vi "SolenoidTest.vi"() -> ()   [LabVIEW 2013]
uses:
  <vilib>/Rock Robotics/SystemInterfaces/DIO/FPGA_DIOChannel.ctl
  <vilib>/Rock Robotics/SystemInterfaces/Typedef/FPGA_TypedefDigitalModule.ctl
  <vilib>/Rock Robotics/SystemInterfaces/DIO/FPGA_DIORelayChannel.ctl
  <vilib>/Rock Robotics/WPI/Joystick/WPI_JoystickDeviceEnum.ctl
  <vilib>/Rock Robotics/WPI/Solenoid/WPI_SolenoidChannel.ctl
  Robot_Framework_2014/DoubleSolenoidAction.ctl
  Robot_Framework_2014/SingleSolenoidAction.ctl
  <vilib>/Rock Robotics/WPI/Solenoid/WPI_SolenoidOpenSingle.vi
panel:
  in  "Single?":bool
  # "BUTTON 5\nL1"
  # "BUTTON 6\nR1"
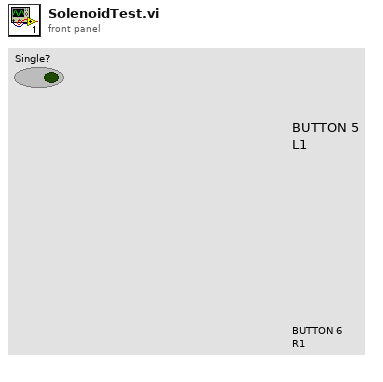
[diagram p1: front panel]
types:
  T1 = typedef "WPI_JoystickDeviceEnum.ctl" = enum16{"USB 1", "USB 2", "USB 3", "USB 4", "Kinect 1", "Kinect 2"}
  T2 = typedef "FPGA_DIORelayChannel.ctl" = enum8{"Relay 1", "Relay 2", "Relay 3", "Relay 4", "Relay 5", "Relay 6", "Relay 7", "Relay 8", "Invalid"}
  T3 = typedef "FPGA_TypedefDigitalModule.ctl" = enum16{"Digital Module 1", "Digital Module 2"}
  T4 = typedef "FPGA_DIOChannel.ctl" = enum8{"DIO 1", "DIO 2", "DIO 3", "DIO 4", "DIO 5", "DIO 6", "DIO 7", "DIO 8", "DIO 9", "DIO 10", "DIO 11", "DIO 12", "DIO 13", "DIO 14", "Invalid"}
  T5 = typedef "WPI_JoystickDevRef.ctl" = cluster{"Device":T1}
  T6 = typedef "DoubleSolenoidAction.ctl" = enum16{"Init", "Middle", "In", "Out"}
  T7 = typedef "WPI_SolenoidChannel.ctl" = enum8{"Solenoid 1", "Solenoid 2", "Solenoid 3", "Solenoid 4", "Solenoid 5", "Solenoid 6", "Solenoid 7", "Solenoid 8", "Invalid"}
  T8 = typedef "SingleSolenoidAction.ctl" = enum16{"Init", "SetState", "Disable"}
  T9 = typedef "WPI_SolenoidDevRef.ctl" = cluster{"DevStatus":errorcluster, "Solenoid Module":T10, "Forward Solenoid Channel":T7, "Reverse Solenoid Channel":T7}
  T10 = typedef "FPGA_TypedefSolenoidModule.ctl" = enum16{"Solenoid Module 1", "Solenoid Module 2"}
  T11 = typedef "WPI_JoystickButtonState.ctl" = cluster{"Button 1":bool, "Button 2":bool, "Button 3":bool, "Button 4":bool, "Button 5":bool, "Button 6":bool, "Button 7":bool, "Button 8":bool, "Button 9":bool, "Button 10":bool, "Button 11":bool, "Button 12":bool}
  T12 = typedef "WPI_CompressorDevRef.ctl" = cluster{"DevStatus":errorcluster, "DigitalInputDevRef":T13, "RelayDevRef":T14}
  T13 = typedef "WPI_DigitalInputDevRef.ctl" = cluster{"DevStatus":errorcluster, "DIO Channel":T4, "Digital Module":T3}
  T14 = typedef "WPI_RelayDevRef.ctl" = cluster{"DevStatus":errorcluster, "Relay Channel":T2, "Digital Module":T3, "Relay Direction":T15}
  T15 = typedef "WPI_RelayDirection.ctl" = enum16{"Both directions", "Forward only", "Reverse only"}
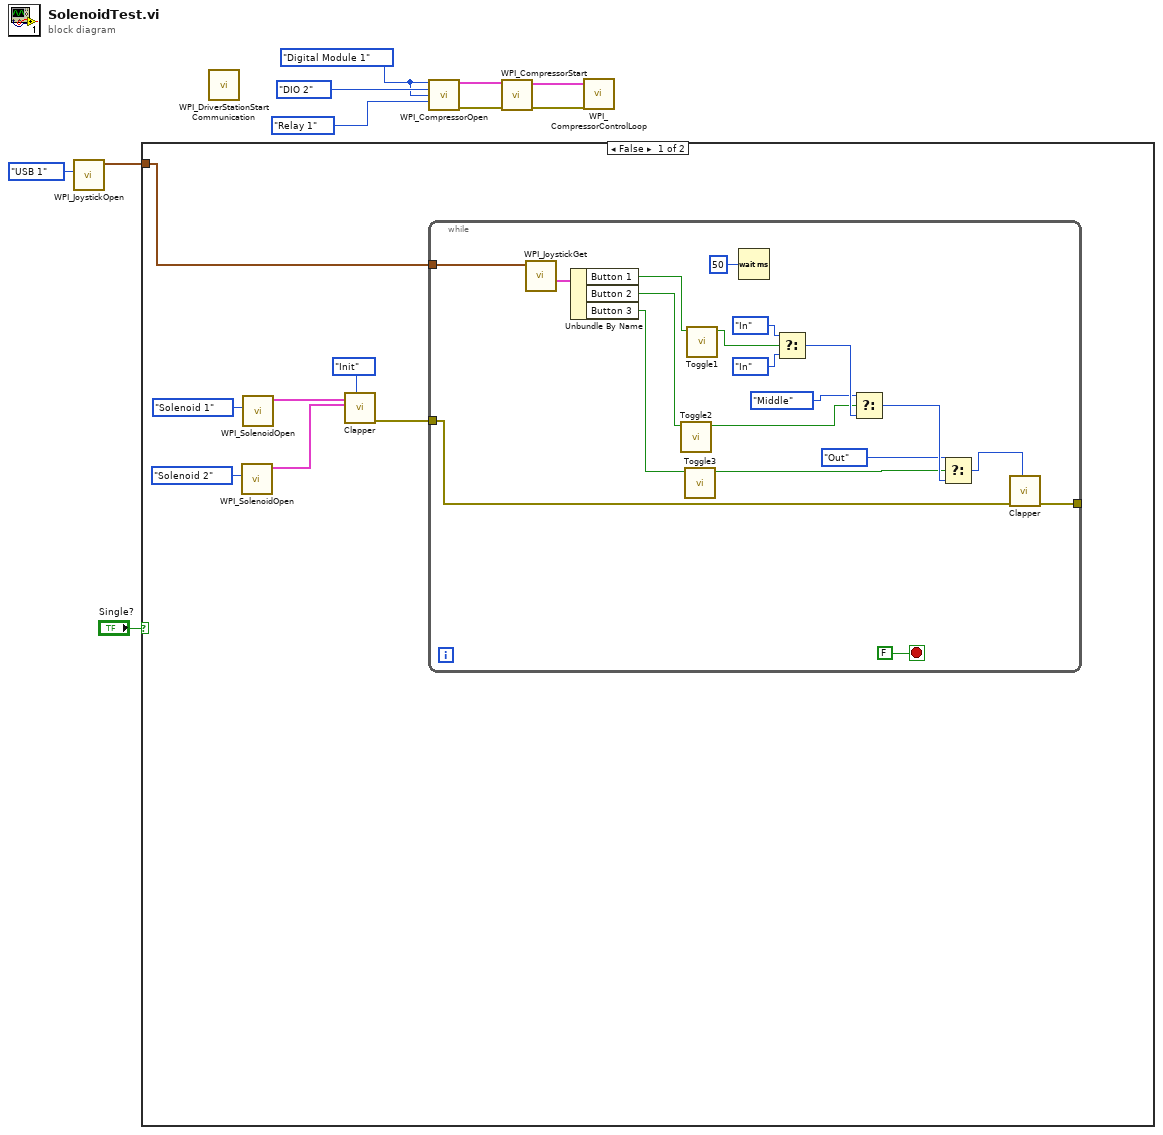
[diagram p0: block diagram]
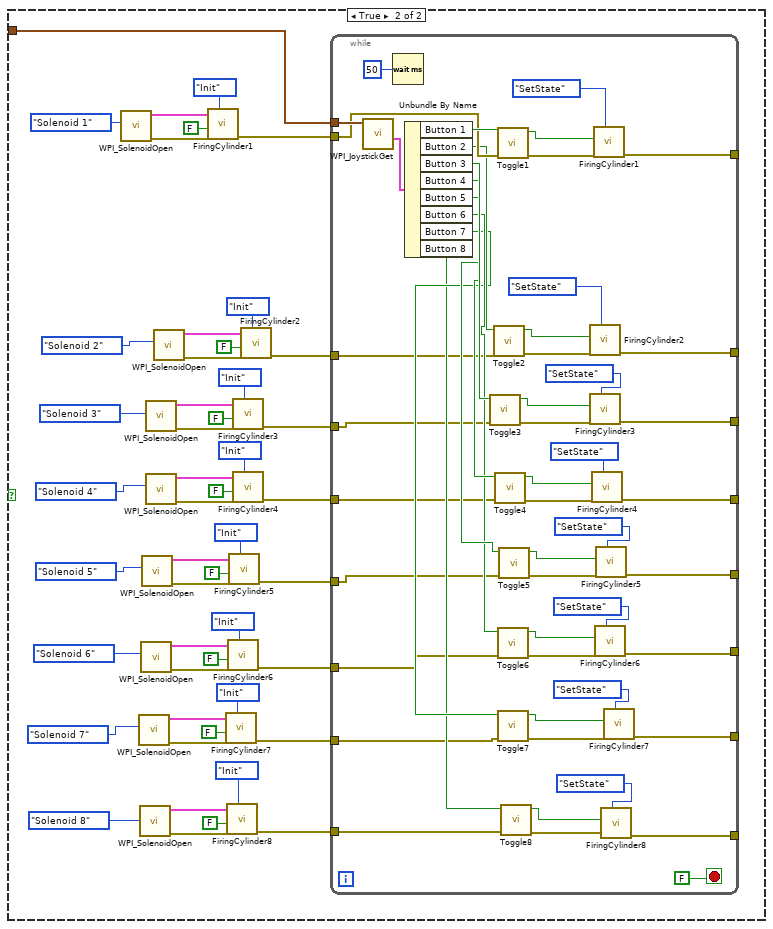
[diagram p2: hidden frame]
diagram:
  w9 = FPGA_TypedefDigitalModule."Digital Module 1" ("Pressure Switch Digital Module (Module 1)")
  n1 = call <vilib>:"WPI_JoystickOpen.vi"("JoystickDevice"=WPI_JoystickDeviceEnum."USB 1") -> ("JoystickDevRef"=w1:T5)  [unwired: 10 in]
  n2 = case shown="False" "Single?" {
    tunnel: w1 -> [w12 w37]
    frame False {
      n3 = call-poly <vilib>:"WPI_SolenoidOpen.vi"("Solenoid Channel"=WPI_SolenoidChannel."Solenoid 2") -> ("SolenoidDevRef"=w14:T9)  [unwired: 9 in, 1 out]
      n4 = call-poly <vilib>:"WPI_SolenoidOpen.vi"("Solenoid Channel"=WPI_SolenoidChannel."Solenoid 1") -> ("SolenoidDevRef"=w15:T9)  [unwired: 9 in, 1 out]
      n5 = call "Clapper.vi"("State"=DoubleSolenoidAction."Init", "Plugged"=w14, "Open"=w15) -> ("Error out"=w13:errorcluster)  [unwired: 8 in]
      n6 = while {
        tunnel: w13 -> [w19]
        tunnel: w12 -> [w34]
        tunnel: [w18] -> _
        stop <- FALSE stop-if-true
        n7 = call <vilib>:"WPI_JoystickGet.vi"("JoystickDevRef"=w34) -> ("Buttons"=w32:T11)  [unwired: 4 in, 2 out]
        n8 = Unbundle By Name(w32) -> ("Button 1"=w31:bool, "Button 2"=w30:bool, "Button 3"=w29:bool)
        n9 = call "Toggle2.vi"("RawInput"=w30) -> ("ToggleState"=w24:bool)  [unwired: 9 in, 1 out]
        n10 = call "Toggle3.vi"("RawInput"=w29) -> ("ToggleState"=w21:bool)  [unwired: 9 in, 1 out]
        n11 = call "Toggle1.vi"("RawInput"=w31) -> ("ToggleState"=w33:bool)  [unwired: 9 in, 1 out]
        n12 = Wait (ms)(milliseconds to wait=u32 50) -> ()  [unwired: 1 out]
        n13 = Select(t=DoubleSolenoidAction."In" ("State"), s=w33, f=DoubleSolenoidAction."In" ("State")) -> (s? t:f=w26:T6)
        n14 = Select(t=DoubleSolenoidAction."Middle" ("State"), s=w24, f=w26) -> (s? t:f=w23:T6)
        n15 = Select(t=DoubleSolenoidAction."Out" ("State"), s=w21, f=w23) -> (s? t:f=w20:T6)
        n16 = call "Clapper.vi"("State"=w20, "Error in"=w19) -> ("Error out"=w18:errorcluster)  [unwired: 9 in]
      }
    }
    frame True {
      n17 = call-poly <vilib>:"WPI_SolenoidOpen.vi"("Solenoid Channel"=WPI_SolenoidChannel."Solenoid 1") -> ("error out"=w81:errorcluster, "SolenoidDevRef"=w82:T9)  [unwired: 9 in]
      n18 = call-poly <vilib>:"WPI_SolenoidOpen.vi"("Solenoid Channel"=WPI_SolenoidChannel."Solenoid 7") -> ("error out"=w61:errorcluster, "SolenoidDevRef"=w60:T9)  [unwired: 9 in]
      n19 = call-poly <vilib>:"WPI_SolenoidOpen.vi"("Solenoid Channel"=WPI_SolenoidChannel."Solenoid 8") -> ("error out"=w56:errorcluster, "SolenoidDevRef"=w57:T9)  [unwired: 9 in]
      n20 = call-poly <vilib>:"WPI_SolenoidOpen.vi"("Solenoid Channel"=WPI_SolenoidChannel."Solenoid 6") -> ("error out"=w62:errorcluster, "SolenoidDevRef"=w63:T9)  [unwired: 9 in]
      n21 = call-poly <vilib>:"WPI_SolenoidOpen.vi"("Solenoid Channel"=WPI_SolenoidChannel."Solenoid 5") -> ("error out"=w68:errorcluster, "SolenoidDevRef"=w67:T9)  [unwired: 9 in]
      n22 = call-poly <vilib>:"WPI_SolenoidOpen.vi"("Solenoid Channel"=WPI_SolenoidChannel."Solenoid 3") -> ("error out"=w76:errorcluster, "SolenoidDevRef"=w75:T9)  [unwired: 9 in]
      n23 = call-poly <vilib>:"WPI_SolenoidOpen.vi"("Solenoid Channel"=WPI_SolenoidChannel."Solenoid 4") -> ("error out"=w69:errorcluster, "SolenoidDevRef"=w70:T9)  [unwired: 9 in]
      n24 = call-poly <vilib>:"WPI_SolenoidOpen.vi"("Solenoid Channel"=WPI_SolenoidChannel."Solenoid 2") -> ("error out"=w77:errorcluster, "SolenoidDevRef"=w78:T9)  [unwired: 9 in]
      n25 = call "FiringCylinder1.vi"("Action"=SingleSolenoidAction."Init", "error in (no error)"=w81, "Default Position"=FALSE, "SolenoidDevRef"=w82) -> ("error out"=w84:errorcluster)  [unwired: 7 in]
      n26 = call "FiringCylinder7.vi"("Action"=SingleSolenoidAction."Init", "error in (no error)"=w61, "Default Position"=FALSE, "SolenoidDevRef"=w60) -> ("error out"=w50:errorcluster)  [unwired: 7 in]
      n27 = call "FiringCylinder8.vi"("Action"=SingleSolenoidAction."Init", "error in (no error)"=w56, "Default Position"=FALSE, "SolenoidDevRef"=w57) -> ("error out"=w49:errorcluster)  [unwired: 7 in]
      n28 = call "FiringCylinder6.vi"("Action"=SingleSolenoidAction."Init", "error in (no error)"=w62, "Default Position"=FALSE, "SolenoidDevRef"=w63) -> ("error out"=w51:errorcluster)  [unwired: 7 in]
      n29 = call "FiringCylinder5.vi"("Action"=SingleSolenoidAction."Init", "error in (no error)"=w68, "Default Position"=FALSE, "SolenoidDevRef"=w67) -> ("error out"=w52:errorcluster)  [unwired: 7 in]
      n30 = call "FiringCylinder3.vi"("Action"=SingleSolenoidAction."Init", "error in (no error)"=w76, "Default Position"=FALSE, "SolenoidDevRef"=w75) -> ("error out"=w54:errorcluster)  [unwired: 7 in]
      n31 = call "FiringCylinder4.vi"("Action"=SingleSolenoidAction."Init", "error in (no error)"=w69, "Default Position"=FALSE, "SolenoidDevRef"=w70) -> ("error out"=w53:errorcluster)  [unwired: 7 in]
      n32 = call "FiringCylinder2.vi"("Action"=SingleSolenoidAction."Init", "error in (no error)"=w77, "Default Position"=FALSE, "SolenoidDevRef"=w78) -> ("error out"=w55:errorcluster)  [unwired: 7 in]
      n33 = while {
        tunnel: w84 -> [w132]
        tunnel: w37 -> [w136]
        tunnel: w55 -> [w118]
        tunnel: w54 -> [w119]
        tunnel: w53 -> [w120]
        tunnel: w52 -> [w121]
        tunnel: w51 -> [w122]
        tunnel: w50 -> [w123]
        tunnel: w49 -> [w124]
        tunnel: [w115] -> _
        tunnel: [w110] -> _
        tunnel: [w108] -> _
        tunnel: [w103] -> _
        tunnel: [w99] -> _
        tunnel: [w95] -> _
        tunnel: [w91] -> _
        tunnel: [w87] -> _
        stop <- FALSE stop-if-true
        n34 = call <vilib>:"WPI_JoystickGet.vi"("JoystickDevRef"=w136) -> ("Buttons"=w135:T11)  [unwired: 4 in, 2 out]
        n35 = Wait (ms)(milliseconds to wait=u32 50) -> ()  [unwired: 1 out]
        n36 = Unbundle By Name(w135) -> ("Button 1"=w134:bool, "Button 2"=w131:bool, "Button 3"=w130:bool, "Button 4"=w129:bool, "Button 5"=w128:bool, "Button 6"=w127:bool, "Button 7"=w126:bool, "Button 8"=w125:bool)
        n37 = call "Toggle3.vi"("error in"=w119, "RawInput"=w130) -> ("error out"=w109:errorcluster, "ToggleState"=w106:bool)  [unwired: 8 in]
        n38 = call "Toggle2.vi"("error in"=w118, "RawInput"=w131) -> ("error out"=w111:errorcluster, "ToggleState"=w112:bool)  [unwired: 8 in]
        n39 = call "Toggle4.vi"("error in"=w120, "RawInput"=w129) -> ("error out"=w104:errorcluster, "ToggleState"=w102:bool)  [unwired: 8 in]
        n40 = call "Toggle1.vi"("error in"=w132, "RawInput"=w134) -> ("error out"=w117:errorcluster, "ToggleState"=w116:bool)  [unwired: 8 in]
        n41 = call "Toggle6.vi"("error in"=w122, "RawInput"=w127) -> ("error out"=w96:errorcluster, "ToggleState"=w94:bool)  [unwired: 8 in]
        n42 = call "Toggle7.vi"("error in"=w123, "RawInput"=w126) -> ("error out"=w92:errorcluster, "ToggleState"=w90:bool)  [unwired: 8 in]
        n43 = call "Toggle5.vi"("error in"=w121, "RawInput"=w128) -> ("error out"=w100:errorcluster, "ToggleState"=w98:bool)  [unwired: 8 in]
        n44 = call "Toggle8.vi"("error in"=w124, "RawInput"=w125) -> ("error out"=w88:errorcluster, "ToggleState"=w86:bool)  [unwired: 8 in]
        n45 = call "FiringCylinder2.vi"("Action"=SingleSolenoidAction."SetState", "error in (no error)"=w111, "Actuate?"=w112) -> ("error out"=w110:errorcluster)  [unwired: 8 in]
        n46 = call "FiringCylinder3.vi"("Action"=SingleSolenoidAction."SetState", "error in (no error)"=w109, "Actuate?"=w106) -> ("error out"=w108:errorcluster)  [unwired: 8 in]
        n47 = call "FiringCylinder4.vi"("Action"=SingleSolenoidAction."SetState", "error in (no error)"=w104, "Actuate?"=w102) -> ("error out"=w103:errorcluster)  [unwired: 8 in]
        n48 = call "FiringCylinder1.vi"("Action"=SingleSolenoidAction."SetState", "error in (no error)"=w117, "Actuate?"=w116) -> ("error out"=w115:errorcluster)  [unwired: 8 in]
        n49 = call "FiringCylinder6.vi"("Action"=SingleSolenoidAction."SetState", "error in (no error)"=w96, "Actuate?"=w94) -> ("error out"=w95:errorcluster)  [unwired: 8 in]
        n50 = call "FiringCylinder5.vi"("Action"=SingleSolenoidAction."SetState", "error in (no error)"=w100, "Actuate?"=w98) -> ("error out"=w99:errorcluster)  [unwired: 8 in]
        n51 = call "FiringCylinder8.vi"("Action"=SingleSolenoidAction."SetState", "error in (no error)"=w88, "Actuate?"=w86) -> ("error out"=w87:errorcluster)  [unwired: 8 in]
        n52 = call "FiringCylinder7.vi"("Action"=SingleSolenoidAction."SetState", "error in (no error)"=w92, "Actuate?"=w90) -> ("error out"=w91:errorcluster)  [unwired: 8 in]
      }
    }
  }
  n53 = call <vilib>:"WPI_DriverStationStart Communication.vi"() -> ()  [unwired: 12 in]
  n54 = call <vilib>:"WPI_CompressorOpen.vi"("Pressure Switch Digital Module (Module 1)"=w9, "Pressure Switch DIO Channel"=FPGA_DIOChannel."DIO 2", "Relay Digital Module (Module 1)"=w9, "Relay Channel"=FPGA_DIORelayChannel."Relay 1") -> ("CompressorDevRef"=w7:T12, "error out"=w6:errorcluster)  [unwired: 10 in]
  n55 = call <vilib>:"WPI_CompressorStart.vi"("error in (no error)"=w6, "CompressorDevRef"=w7) -> ("error out"=w5:errorcluster, "CompressorDevRef"=w4:T12)  [unwired: 8 in]
  n56 = call <vilib>:"WPI_CompressorControlLoop.vi"("error in (no error)"=w5, "CompressorDevRef"=w4) -> ()  [unwired: 10 in]
